vi "Requisitante.vi"() -> ()   [LabVIEW 2018]
uses:
  RxTx/CM_RxTx.lvclass
panel:
  out "error out":errorcluster
  in  "Queue RX":refnum<class "CM_RxTx.lvclass">
  out "Reply":string
  in  "Request":string
  in  "send":bool
  in  "stop":bool
  # "REQ endpoint"
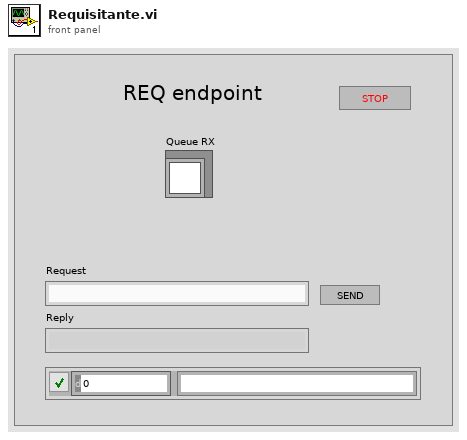
[diagram p1: front panel]
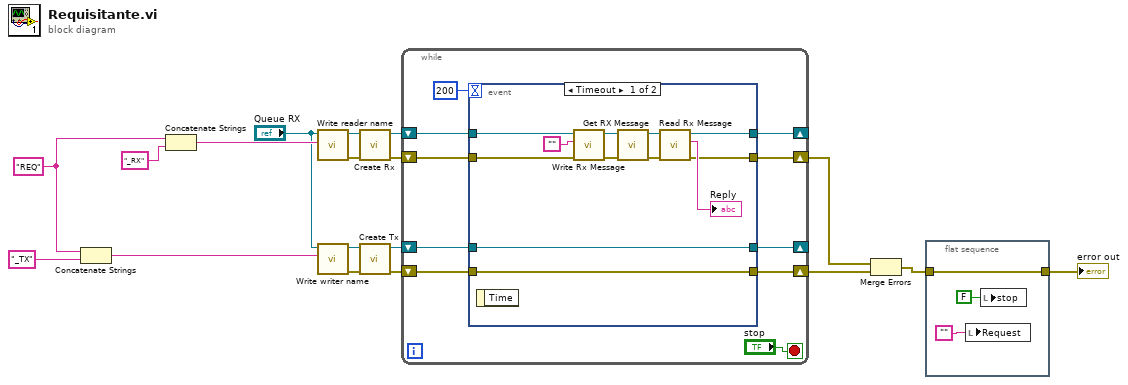
[diagram p0: block diagram]
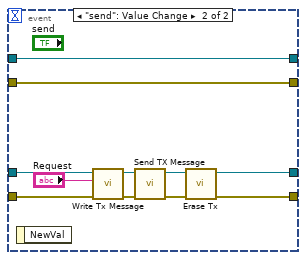
[diagram p2: hidden frame]
diagram:
  w1 = "REQ"
  n1 = Concatenate Strings(w1, "_TX" ("string")) -> (w3:string)
  n2 = Concatenate Strings(w1, "_RX" ("string")) -> (w4:string)
  n3 = call-dynamic "Write reader name.vi"("RX name"=w4, "RxTx in"="Queue RX") -> ("error out"=w13:errorcluster, "RxTx out"=w14:refnum<class "CM_RxTx.lvclass">)  [unwired: 8 in]
  n4 = call-dynamic "Write writer name.vi"("Tx name"=w3, "RxTx in"="Queue RX") -> ("error out"=w12:errorcluster, "RxTx out"=w15:refnum<class "CM_RxTx.lvclass">)  [unwired: 8 in]
  n5 = call "Create Rx.vi"("error in (no error)"=w13, "RxTx in"=w14) -> ("error out"=w10:errorcluster, "RxTx out"=w16:refnum<class "CM_RxTx.lvclass">)  [unwired: 8 in]
  n6 = call "Create Tx.vi"("error in (no error)"=w12, "RxTx in"=w15) -> ("error out"=w11:errorcluster, "RxTx out"=w18:refnum<class "CM_RxTx.lvclass">)  [unwired: 8 in]
  n7 = while {
    shift-right: [w27] -> _
    shift-left: w18 -> [w28]
    shift-right: [w23] -> _
    shift-left: w16 -> [w24]
    shift-right: [w21] -> w8
    shift-left: w11 -> [w22]
    shift-right: [w19] -> w9
    shift-left: w10 -> [w20]
    stop <- "stop" stop-if-true
    n8 = event shown="[0] Timeout" {
      selector: _ -> [_ _]
      dyn-events: _ -> [_ _]
      timeout: 200 -> [_ _]
      tunnel: w28 -> [w40 w51]
      tunnel: [w40 w41] -> w27
      tunnel: w24 -> [w36 w47]
      tunnel: [w34 w47] -> w23
      tunnel: w22 -> [w31 w46]
      tunnel: [w31 w42] -> w21
      tunnel: w20 -> [w30 w45]
      tunnel: [w29 w45] -> w19
      event Timeout {
        n9 = event-data() -> ()  [unwired: 1 in, 1 out]
        n10 = call "Write Rx Message.vi"("error in (no error)"=w30, "Rx Message"="", "RxTx in"=w36) -> ("error out"=w33:errorcluster, "RxTx out"=w35:refnum<class "CM_RxTx.lvclass">)  [unwired: 7 in]
        n11 = call "Get RX Message.vi"("error in (no error)"=w33, "RxTx in"=w35) -> ("error out"=w37:errorcluster, "RxTx out"=w39:refnum<class "CM_RxTx.lvclass">)  [unwired: 7 in, 1 out]
        n12 = call "Read Rx Message.vi"("error in (no error)"=w37, "RxTx in"=w39) -> ("error out"=w29:errorcluster, "Rx Message"=→"Reply":string, "RxTx out"=w34:refnum<class "CM_RxTx.lvclass">)  [unwired: 7 in]
      }
      event "send": Value Change {
        n13 = event-data() -> ()  [unwired: 1 in, 1 out]
        n14 = call "Write Tx Message.vi"("error in (no error)"=w46, "Tx Message"="Request", "RxTx in"=w51) -> ("error out"=w48:errorcluster, "RxTx out"=w49:refnum<class "CM_RxTx.lvclass">)  [unwired: 7 in]
        n15 = call "Send TX Message.vi"("error in (no error)"=w48, "RxTx in"=w49) -> ("error out"=w43:errorcluster, "RxTx out"=w44:refnum<class "CM_RxTx.lvclass">)  [unwired: 8 in]
        n16 = call "Erase Tx.vi"("error in (no error)"=w43, "RxTx in"=w44) -> ("error out"=w42:errorcluster, "RxTx out"=w41:refnum<class "CM_RxTx.lvclass">)  [unwired: 8 in]
      }
    }
  }
  n17 = Merge Errors(w9, w8) -> (w6:errorcluster)
  n18 = flat-sequence {
    tunnel: w6 -> [w54]
    tunnel: [w54] -> w5
    frame #0 {
      n19 = local write "Request"("") -> ()
      n20 = local write "stop"(FALSE ("stop")) -> ()
    }
  }
  "error out" <- w5
